vi "DrawEllipseOnImageGreyscale.vi"(4 "Thickness (Default: 1)":i32=1, 5 "Ellipse Angles (Default: No rotation & full)":T2={"Rotation"=0.0, "Start"=0.0, "Stop"=360.0}, 6 "Colour":u8=255, 7 "OpenCV Line Type (Default LINE_8)":T4=enum."LINE_8", 8 "error in (no error)":errorcluster, 9 "Axes":T1, 10 "Centre":T3, 11 "Greyscale Image":refnum<data-value>) -> (0 "error out":errorcluster, 3 "Greyscale Image (Duplicate)":refnum<data-value>)   [LabVIEW 2020, in "g_ar_toolkit.image.lvlib"]
uses:
  g_ar_toolkit.image.lvlib
  Line Type.ctl
  g_ar_toolkit.common/Image Point (Integer).ctl
  Ellipse Angles.ctl
  g_ar_toolkit.common/Image Size (Integer).ctl
  <vilib>/Utility/error.llb/Error Cluster From Error Code.vi
  eaaaec5c-60e1-4320-b5ad-f9d454208055.vi
  g_ar_toolkit.common/g_ar_toolkit_common.lvlib
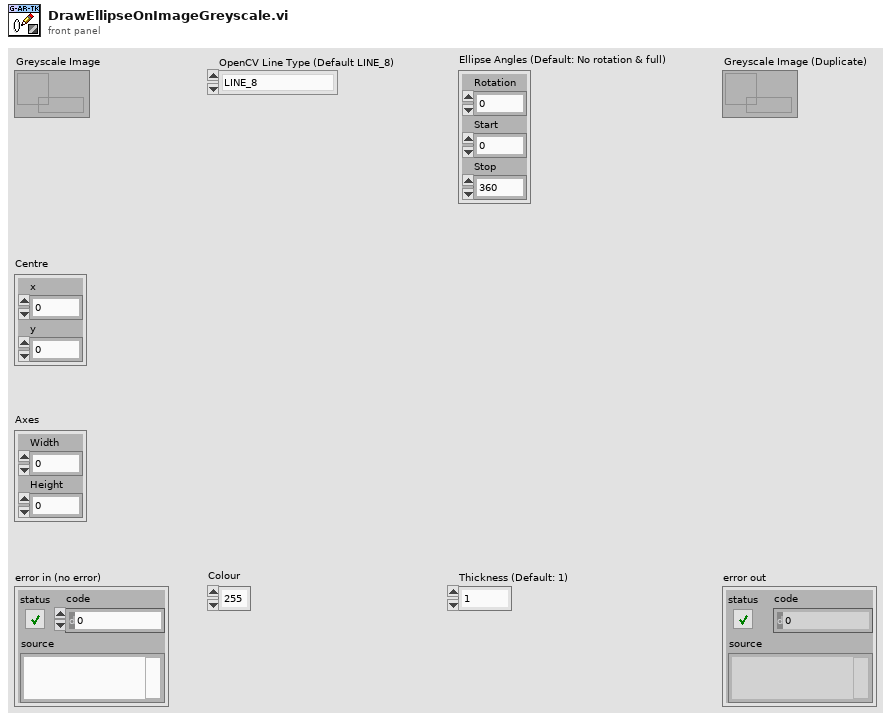
[diagram p1: front panel]
types:
  T1 = typedef "g_ar_toolkit_common.lvlib/Image Size (Integer).ctl" = cluster{"Width":u16, "Height":u16}
  T2 = typedef "g_ar_toolkit.image.lvlib/Ellipse Angles.ctl" = cluster{"Rotation":dbl, "Start":dbl, "Stop":dbl}
  T3 = typedef "g_ar_toolkit_common.lvlib/Image Point (Integer).ctl" = cluster{"x":i32, "y":i32}
  T4 = typedef "g_ar_toolkit.image.lvlib/Line Type.ctl" = enum8{"FILLED", "LINE_4", "LINE_8", "LINE_AA"}
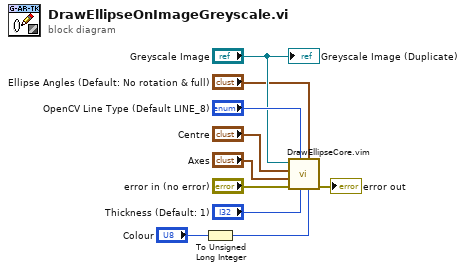
[diagram p0: block diagram]
diagram:
  n1 = To Unsigned Long Integer(number="Colour") -> (unsigned 32bit integer=w5:u32)
  n2 = call "DrawEllipseCore.vim"("Colour"=w5, "Ellipse Angles"="Ellipse Angles (Default: No rotation & full)", "Thickness"="Thickness (Default: 1)", "OpenCV Line Type"="OpenCV Line Type (Default LINE_8)", "error in (no error)"="error in (no error)", "Axes"="Axes", "Centre"="Centre", "Src"="Greyscale Image") -> ("error out"=→"error out":errorcluster)  [unwired: 3 in]
  "Greyscale Image (Duplicate)" <- "Greyscale Image"
